vi "Has Left.vi"(8 "error in (no error)":errorcluster, 11 "SnailNum in":refnum<class "SnailNum.lvclass">) -> (0 "error out":errorcluster, 2 "Has Left":bool, 3 "SnailNum out":refnum<class "SnailNum.lvclass">)   [LabVIEW 2020, in "SnailNum.lvclass"]
uses:
  SnailNum.lvclass
  SnailNum.lvclass/SnailNum.ctl
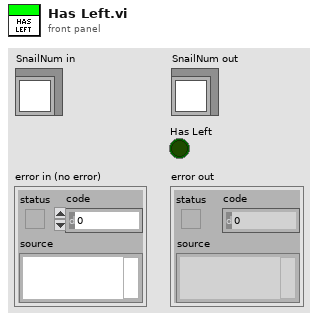
[diagram p1: front panel]
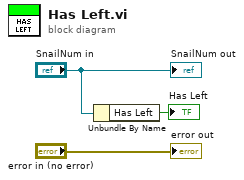
[diagram p0: block diagram]
diagram:
  n1 = Unbundle By Name("SnailNum in") -> ("Has Left"=→"Has Left":bool)
  "error out" <- "error in (no error)"
  "SnailNum out" <- "SnailNum in"
